vi "StringLaserTransmitter.vi"() -> ()   [LabVIEW 2012]
panel:
  in  "milliseconds to wait":u32
  in  "width (-)":i32
  out "boolean integer string":string
  in  "number":i32
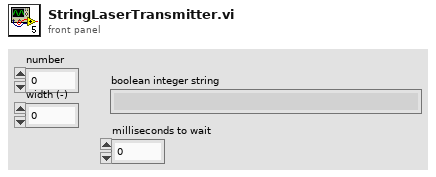
[diagram p1: front panel]
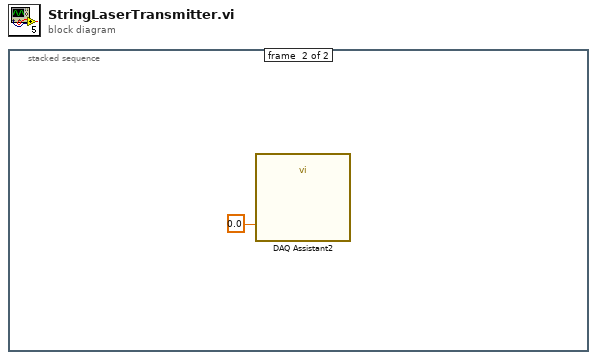
[diagram p0: block diagram]
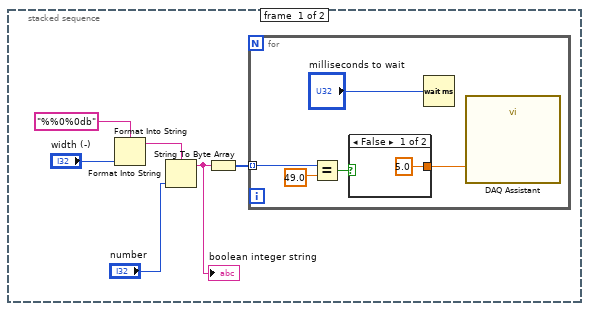
[diagram p2: hidden frame]
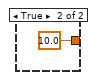
[diagram p3: hidden frame]
diagram:
  n1 = stacked-sequence {
    frame #0 {
      n2 = Format Into String(format string="%%0%0db", "width (-)") -> (resulting string=w6:string)  [unwired: 2 in, 1 out]
      n3 = Format Into String(format string=w6, "number") -> (resulting string=w3:string)  [unwired: 2 in, 1 out]
      "boolean integer string" <- w3
      n4 = String To Byte Array(string=w3) -> (unsigned byte array=w2:u8[])
      n5 = for {
        tunnel: w2 -> [w9] mode=indexing
        n6 = Equal?(x=w9, y=49.0) -> (x = y?=w11:bool)
        n7 = case shown="False" w11 {
          tunnel: [5.0 ("data") 10.0 ("data")] -> w8
          frame False {
          }
          frame True {
          }
        }
        n8 = Wait (ms)(milliseconds to wait="milliseconds to wait") -> ()  [unwired: 1 out]
        n9 = call "DAQ Assistant"("data"=w8) -> ()  [unwired: 17 in, 2 out]
      }
    }
    frame #1 {
      n10 = call "DAQ Assistant2"("data"=0.0) -> ()  [unwired: 17 in, 2 out]
    }
  }
